vi "WZ5005E-Read.vi"(8 "error in":errorcluster caption="错误输入（无错误）", 10 "地址":string="02", 11 "MyIndex":u8) -> (0 "error out":errorcluster, 1 "输出功率":dbl, 2 "输出电流":dbl, 3 "输出电压":dbl, 4 "输入电压":dbl)   [LabVIEW 2015, in "WZ5005E.lvlib"]
uses:
  WZ5005E.lvlib
  <vilib>/Instr/_visa.llb/VISA Configure Serial Port (Instr).vi
panel:
  out "VISA":refnum<visa-resource-name>
  out "Read":string
  out "Send":string
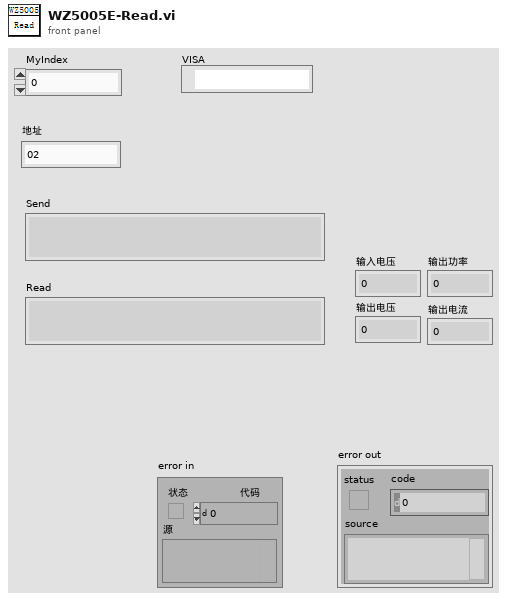
[diagram p1: front panel]
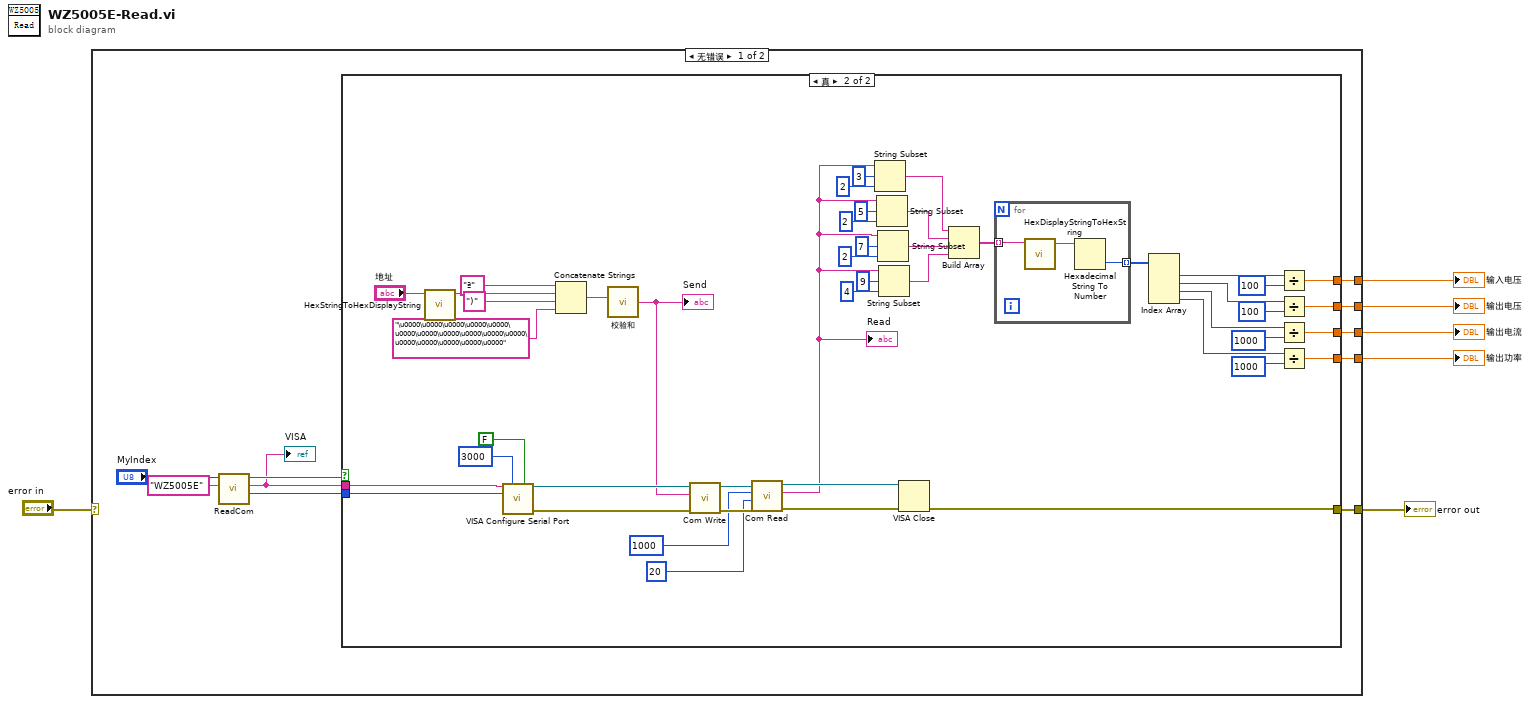
[diagram p0: block diagram]
diagram:
  n1 = case shown="无错误" "error in" {
    selector: "error in" -> [_ w67]
    tunnel: [w16 w67] -> w6
    tunnel: [w10 _] -> w4
    tunnel: [w9 _] -> w3
    tunnel: [w8 _] -> w2
    tunnel: [w7 _] -> w1
    frame No Error {
      n2 = call "ReadCom.vi"("仪器名称"="WZ5005E", "MyIndex"="MyIndex") -> ("Baudrate"=w11:i32, "COM"=w12:string, "OK?"=w13:bool)  [unwired: 7 in]
      "VISA" <- w12
      n3 = case shown="真" w13 {
        tunnel: [_ w63] -> w16
        tunnel: w12 -> [_ w62]
        tunnel: w11 -> [_ w61]
        tunnel: [_ w20] -> w10
        tunnel: [_ w19] -> w9
        tunnel: [_ w18] -> w8
        tunnel: [_ w17] -> w7
        frame False {
        }
        frame True {
          n4 = call "HexStringToHexDisplayString.vi"("正常显示HEX字符串"="地址") -> ("HEX显示字符串"=w49:string)  [unwired: 10 in]
          n5 = call-poly "VISA Configure Serial Port"("VISA resource name"=w62, "timeout (10sec)"=u32 3000, "Enable Termination\nChar (T)"=FALSE ("Enable Termination\nChar (T)"), "baud rate (9600)"=w61) -> ("VISA resource name out"=w59:refnum<visa-resource-name>, "error out"=w58:errorcluster)  [unwired: 10 in]
          n6 = Concatenate Strings("ª", w49, ")", "\u0000\u0000\u0000\u0000\u0000\u0000\u0000\u0000\u0000\u0000\u0000\u0000\u0000\u0000\u0000\u0000") -> (w44:string)
          n7 = call "校验和.vi"("输入（Hex）"=w44) -> ("输出"=w45:string)
          "Send" <- w45
          n8 = call "Com Write.vi"("错误输入（无错误）"=w58, "Wbuff"=w45, "VISA In"=w59) -> ("错误输出"=w56:errorcluster, "VISA Out"=w57:refnum<visa-resource-name>)  [unwired: 6 in, 1 out]
          n9 = call "Com Read.vi"("错误输入（无错误）"=w56, "num"=u32 20, "超时"=u32 1000, "VISA In"=w57) -> ("错误输出"=w55:errorcluster, "buff"=w21:string, "VISA Out"=w54:refnum<visa-resource-name>)  [unwired: 4 in, 1 out]
          "Read" <- w21
          n10 = String Subset(string=w21, offset (0)=3 ("偏移量(0)"), length (rest)=2 ("长度（剩余）")) -> (substring=w30:string)
          n11 = String Subset(string=w21, offset (0)=5 ("偏移量(0)"), length (rest)=2 ("长度（剩余）")) -> (substring=w31:string)
          n12 = String Subset(string=w21, offset (0)=7 ("偏移量(0)"), length (rest)=2 ("长度（剩余）")) -> (substring=w32:string)
          n13 = String Subset(string=w21, offset (0)=9 ("偏移量(0)"), length (rest)=4 ("长度（剩余）")) -> (substring=w33:string)
          n14 = VISA Close(VISA resource name=w54, error in (no error)=w55) -> (error out=w63:errorcluster)
          n15 = Build Array(w30, w31, w32, w33) -> (w34:string[])
          n16 = for {
            tunnel: w34 -> [w65] mode=indexing
            tunnel: [w66] -> w35 mode=indexing
            n17 = call "HexDisplayStringToHexString.vi"("HEX显示字符串"=w65) -> ("正常显示HEX字符串"=w64:string)  [unwired: 10 in]
            n18 = Hexadecimal String To Number(string=w64) -> (number=w66:u32)  [unwired: 2 in, 1 out]
          }
          n19 = Index Array(array=w35) -> (element #1=w36:u32, element #2=w38:u32, element #3=w40:u32, element #4=w43:u32)  [unwired: 4 in]
          n20 = Divide(x=w36, y=u32 100) -> (x/y=w20:dbl)
          n21 = Divide(x=w38, y=u32 100) -> (x/y=w19:dbl)
          n22 = Divide(x=w40, y=u32 1000) -> (x/y=w18:dbl)
          n23 = Divide(x=w43, y=u32 1000) -> (x/y=w17:dbl)
        }
      }
    }
    frame Error {
    }
  }
  "error out" <- w6
  "输入电压" <- w4
  "输出电压" <- w3
  "输出电流" <- w2
  "输出功率" <- w1
